vi "3.4.vi"() -> ()   [LabVIEW 2015]
panel:
  out "年龄":dbl
  out "专业":string
  out "名族":string
  out "性别":string
  out "姓名":string
  in  "簇":T1
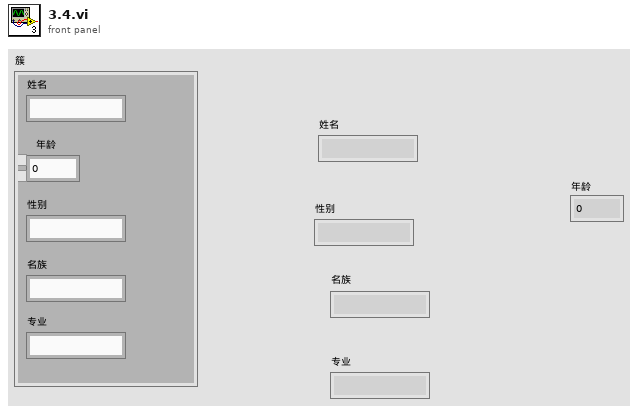
[diagram p1: front panel]
types:
  T1 = cluster{"年龄":dbl, "姓名":string, "性别":string, "名族":string, "专业":string}
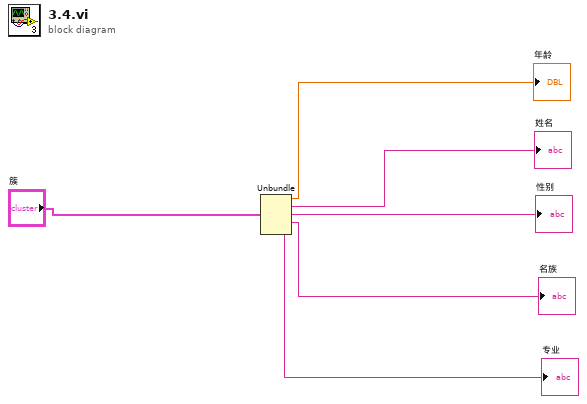
[diagram p0: block diagram]
diagram:
  n1 = Unbundle("簇") -> ("年龄"=→"年龄":dbl, "姓名"=→"姓名":string, "性别"=→"性别":string, "名族"=→"名族":string, "专业"=→"专业":string)
